vi "Initialize kinect systems.vi"(6 "Video and Depth config":T6={"Video Resolution"=enum."FREENECT_RESOLUTION_LOW", "Video Format"=enum."FREENECT_VIDEO_RGB", "Depth Format"=enum."FREENECT_DEPTH_11BIT", "Depth Resolution"=enum."FREENECT_RESOLUTION_MEDIUM"}, 8 "error in (no error)":errorcluster, 9 "Led Option":T7, 10 "tilt degree":i32, 11 "Log Level":T1) -> (0 "error out":errorcluster, 1 "Kinect Handle":i64, 2 "result":i32, 3 "Video Handle out":i64)   [LabVIEW 2015]
uses:
  subVIs/Led Control.ctl
  subVIs/Video Resolution Control.ctl
  subVIs/Video Format Control.ctl
  subVIs/Depth Format Control.ctl
  subVIs/Depth Resolution Control.ctl
  subVIs/Log Level Control.ctl
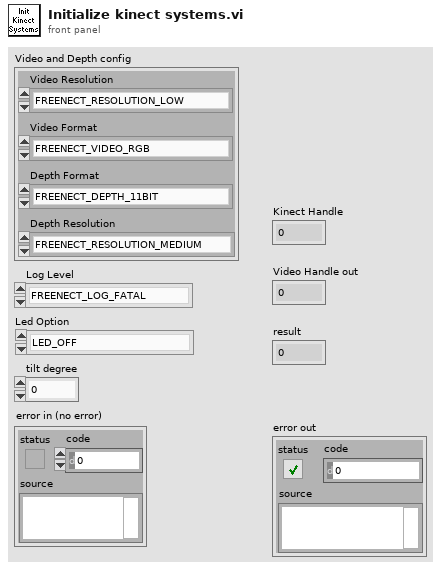
[diagram p1: front panel]
types:
  T1 = typedef "Log Level Control.ctl" = enum32{"FREENECT_LOG_FATAL", "FREENECT_LOG_ERROR", "FREENECT_LOG_WARNING", "FREENECT_LOG_NOTICE", "FREENECT_LOG_INFO", "FREENECT_LOG_DEBUG", "FREENECT_LOG_SPEW", "FREENECT_LOG_FLOOD"}
  T2 = typedef "Video Resolution Control.ctl" = enum32{"FREENECT_RESOLUTION_LOW", "FREENECT_RESOLUTION_MEDIUM", "FREENECT_RESOLUTION_HIGH"}
  T3 = typedef "Video Format Control.ctl" = enum32{"FREENECT_VIDEO_RGB", "FREENECT_VIDEO_BAYER", "FREENECT_VIDEO_IR_8BIT", "FREENECT_VIDEO_IR_10BIT", "FREENECT_VIDEO_IR_10BIT_PACKED", "FREENECT_VIDEO_YUV_RGB", "FREENECT_VIDEO_YUV_RAW"}
  T4 = typedef "Depth Format Control.ctl" = enum32{"FREENECT_DEPTH_11BIT", "FREENECT_DEPTH_10BIT", "FREENECT_DEPTH_11BIT_PACKED", "FREENECT_DEPTH_10BIT_PACKED", "FREENECT_DEPTH_REGISTERED", "FREENECT_DEPTH_MM"}
  T5 = typedef "Depth Resolution Control.ctl" = enum16{"FREENECT_RESOLUTION_TINY", "FREENECT_RESOLUTION_LOW", "FREENECT_RESOLUTION_MEDIUM"}
  T6 = cluster{"Video Resolution":T2, "Video Format":T3, "Depth Format":T4, "Depth Resolution":T5}
  T7 = typedef "Led Control.ctl" = enum32{"LED_OFF", "LED_GREEN", "LED_RED", "LED_YELLOW", "LED_BLINK_GREEN", "LED_BLINK_GREEN2", "LED_BLINK_RED_YELLOW"}
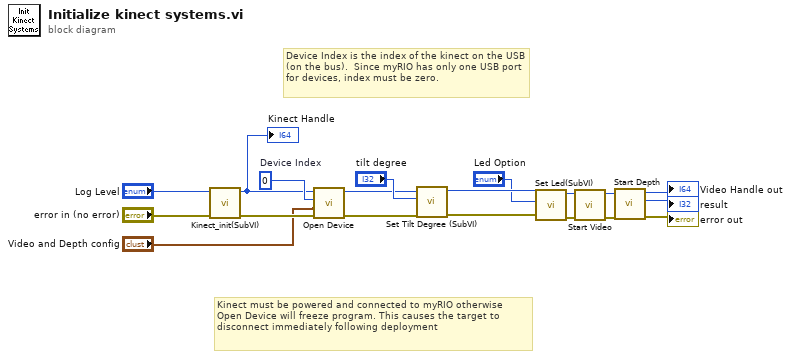
[diagram p0: block diagram]
diagram:
  w15 = 0  # Device Index
  # "Device Index is the index of the kinect on the USB (on the bus).  Since myRIO has only one USB port for devices, index must be zero."
  # "Kinect must be powered and connected to myRIO otherwise Open Device will freeze program. This causes the target to disconnect immediately following deployment"
  n1 = call "Kinect_init(SubVI).vi"("error in (no error)"="error in (no error)", "log_level"="Log Level") -> ("error out"=w17:errorcluster, "Context_handle"=w14:i64)  [unwired: 8 in]
  "Kinect Handle" <- w14
  n2 = call "Open Device.vi"("error in (no error)"=w17, "input cluster"="Video and Depth config", "device index"=w15, "Context_handle"=w14) -> ("error out"=w13:errorcluster, "handle"=w11:i64)  [unwired: 6 in]
  n3 = call "Set Tilt Degree (SubVI).vi"("handle in"=w11, "degree"="tilt degree", "error in (no error)"=w13) -> ("handle out"=w9:i64, "error out"=w10:errorcluster)  [unwired: 6 in]
  n4 = call "Set Led(SubVI).vi"("error in (no error)"=w10, "Led Option"="Led Option", "handle in"=w9) -> ("error out"=w4:errorcluster, "handle out"=w2:i64)  [unwired: 7 in]
  n5 = call "Start Video.vi"("error in (no error)"=w4, "handle in"=w2) -> ("error out"=w3:errorcluster, "handle out"=w1:i64)  [unwired: 7 in, 1 out]
  n6 = call "Start Depth.vi"("error in (no error)"=w3, "handle in"=w1) -> ("error out"=→"error out":errorcluster, "result"=→"result":i32, "handle out"=→"Video Handle out":i64)  [unwired: 7 in]
